vi "ConvertBlockDiagram.vi"(4 "filename":string="BlockDiagram.py", 5 "Source Directory":path, 6 "error in":errorcluster, 9 "VI Interpreter":refnum<class "VI Interpreter.lvclass">) -> (0 "error out":errorcluster, 2 "SubVIs":variant, 3 "VI Interpreter out":refnum<class "VI Interpreter.lvclass">)   [LabVIEW 2014, in "PyConvBD.lvclass"]
uses:
  PyConvBD.lvclass
  VI Interpreter/Classes/VI Interpreter/VI Interpreter.lvclass
  PyConvBD.lvclass/PyConvBD.ctl
  Parsing/Python Functions.lvlib
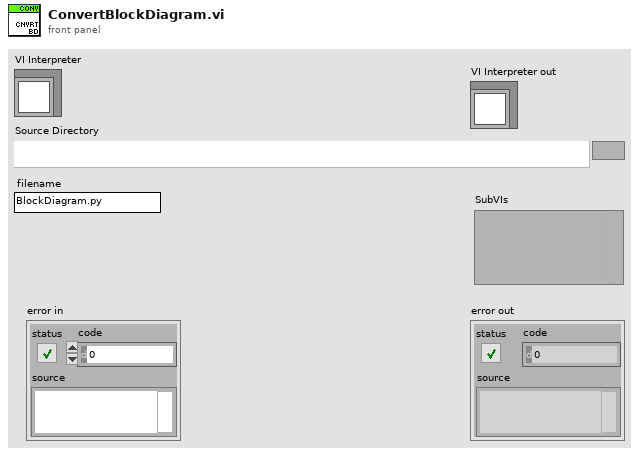
[diagram p1: front panel]
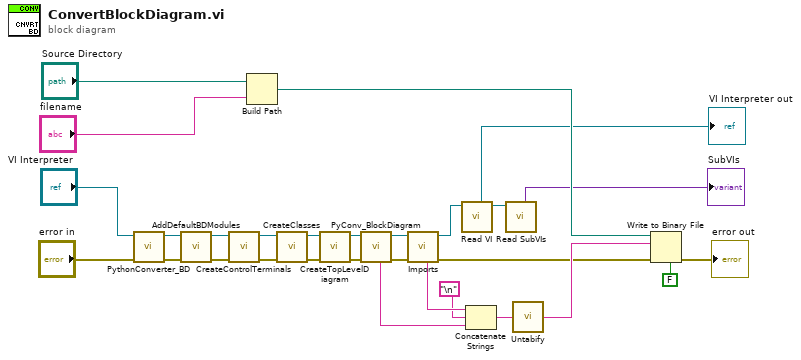
[diagram p0: block diagram]
diagram:
  n1 = call "PythonConverter_BD.vi"("error in"="error in", "VI Interpreter in"="VI Interpreter") -> ("error out"=w23:errorcluster, "PythonConverter_BD out"=w24:refnum<class "PyConvBD.lvclass">)  [unwired: 6 in]
  n2 = call "AddDefaultBDModules.vi"("error in"=w23, "PythonConverter_BD in"=w24) -> ("error out"=w4:errorcluster, "PythonConverter_BD out"=w6:refnum<class "PyConvBD.lvclass">)  [unwired: 8 in]
  n3 = call "CreateControlTerminals.vi"("error in"=w4, "PythonConverter_BD in"=w6) -> ("error out"=w3:errorcluster, "PythonConverter_BD out"=w5:refnum<class "PyConvBD.lvclass">)  [unwired: 8 in]
  n4 = Build Path(base path="Source Directory", name or relative path="filename") -> (appended path=w26:path)
  n5 = call "CreateClasses.vi"("error in"=w3, "PythonConverter_BD in"=w5) -> ("error out"=w21:errorcluster, "PythonConverter_BD out"=w22:refnum<class "PyConvBD.lvclass">)  [unwired: 8 in]
  n6 = call "CreateTopLevelDiagram.vi"("error in"=w21, "PythonConverter_BD in"=w22) -> ("error out"=w29:errorcluster, "PythonConverter_BD out"=w20:refnum<class "PyConvBD.lvclass">)  [unwired: 8 in]
  n7 = call "PyConv_BlockDiagram.vi"("error in"=w29, "PythonConverter_BD in"=w20) -> ("error out"=w18:errorcluster, "PythonConverter_BD out"=w19:refnum<class "PyConvBD.lvclass">, "BlockDiagram"=w7:string)  [unwired: 5 in]
  n8 = call "Imports.vi"("error in"=w18, "PythonConverter_BD in"=w19) -> ("error out"=w15:errorcluster, "PythonConverter_BD out"=w14:refnum<class "PyConvBD.lvclass">, "imports"=w28:string)  [unwired: 5 in]
  n9 = call "Read VI.vi"("PythonConverter_BD in"=w14) -> ("PythonConverter_BD out"=w2:refnum<class "PyConvBD.lvclass">, "VI Interpreter"=→"VI Interpreter out":refnum<class "VI Interpreter.lvclass">)  [unwired: 7 in]
  n10 = Concatenate Strings(w28, "\n", w7) -> (w25:string)
  n11 = call "Read SubVIs.vi"("PyConvBD in"=w2) -> ("SubVIs"=→"SubVIs":variant)  [unwired: 7 in, 1 out]
  n12 = call "Untabify.vi"("string in"=w25) -> ("string out"=w16:string)  [unwired: 1 in]
  n13 = Write to Binary File(file (use dialog)=w26, data=w16, error in=w15, 5:FALSE ("prepend array or string size? (T)")) -> (error out=→"error out":errorcluster)  [unwired: 2 in, 2 out]
